vi "Read Status.vi"(8 "error in (no error)":errorcluster, 10 "Source Name (0: Channel 1)":i32(ring) items=["Channel 1", "Channel 2", "Channel 3", "Channel 4", "Common 1", "Common 2", "Differential 1", "Differential 2", "Function 1", "Function 2", "Function 3", "Function 4", "Function 5", "Function 6", "Function 7", "Function 8", "Function 9", "Function 10", "Function 11", "Function 12", "Function 13", "Function 14", "Function 15", "Function 16", "Histogram", "Memory 1", "Memory 2", "Memory 3", "Memory 4", "Clock", "MTRend", "MSPecturm", "Equalized", "Bus 1", "Bus 2", "Bus 3", "Bus 4", "Digital 0", "Digital 1", "Digital 2", "Digital 3", "Digital 4", "Digital 5", "Digital 6", "Digital 7", "Digital 8", "Digital 9", "Digital 10", "Digital 11", "Digital 12", "Digital 13", "Digital 14", "Digital 15", "Pod 1", "Pod 2"], 11 "VISA resource name":refnum<visa-resource-name>) -> (0 "error out":errorcluster, 2 "Source Status (T: ON)":bool=TRUE, 3 "VISA resource name out":refnum<visa-resource-name>)   [LabVIEW 2020, in "Agilent 90000 Series.lvlib"]
doc: "Queries whether the specified channel, function, wmemory, histogram, measurement trend, measurement spectrum, or equalized waveform is on or off."
uses:
  Agilent 90000 Series.lvlib
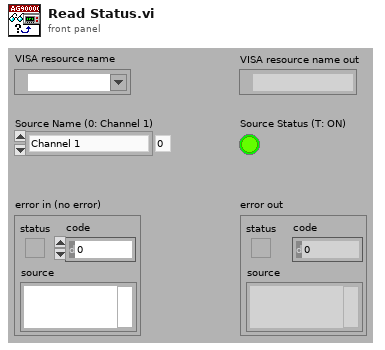
[diagram p1: front panel]
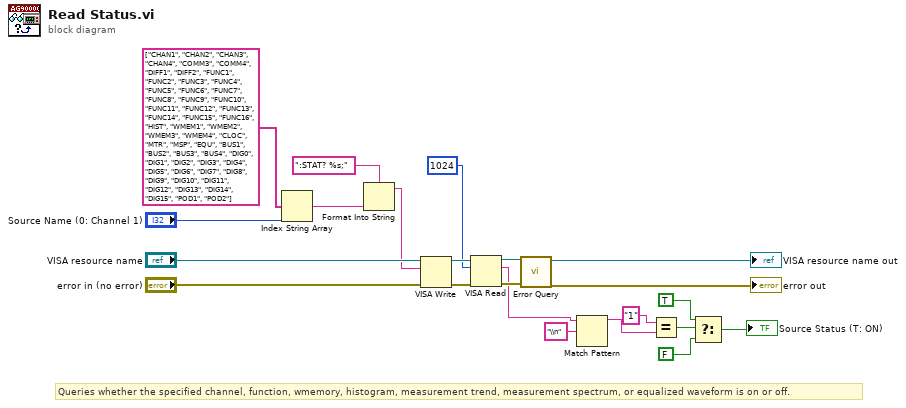
[diagram p0: block diagram]
diagram:
  # "Queries whether the specified channel, function, wmemory, histogram, measurement trend, measurement spectrum, or equalized waveform is on or off."
  n1 = Index String Array(1:"Source Name (0: Channel 1)", 2:string[] ["CHAN1", "CHAN2", "CHAN3", "CHAN4", "COMM3", "COMM4", "DIFF1", "DIFF2", "FUNC1", "FUNC2", "FUNC3", "FUNC4", "FUNC5", "FUNC6", "FUNC7", "FUNC8", "FUNC9", "FUNC10", "FUNC11", "FUNC12", "FUNC13", "FUNC14", "FUNC15", "FUNC16", "HIST", "WMEM1", "WMEM2", "WMEM3", "WMEM4", "CLOC", "MTR", "MSP", "EQU", "BUS1", "BUS2", "BUS3", "BUS4", "DIG0", "DIG1", "DIG2", "DIG3", "DIG4", "DIG5", "DIG6", "DIG7", "DIG8", "DIG9", "DIG10", "DIG11", "DIG12", "DIG13", "DIG14", "DIG15", "POD1", "POD2"] ("string array")) -> (0:w15:string)  [unwired: 1 in]
  n2 = Format Into String(format string=":STAT? %s;", w15) -> (resulting string=w14:string)  [unwired: 2 in, 1 out]
  n3 = VISA Write(VISA resource name="VISA resource name", write buffer=w14, error in (no error)="error in (no error)") -> (VISA resource name out=w13:refnum<visa-resource-name>, error out=w12:errorcluster)  [unwired: 1 out]
  n4 = VISA Read(VISA resource name=w13, byte count=u32 1024, error in (no error)=w12) -> (VISA resource name out=w11:refnum<visa-resource-name>, read buffer=w3:string, error out=w10:errorcluster)  [unwired: 1 out]
  n5 = call "Error Query.vi"("error in (no error)"=w10, "VISA resource name"=w11) -> ("error out"=→"error out":errorcluster, "VISA resource name out"=→"VISA resource name out":refnum<visa-resource-name>)  [unwired: 6 in, 2 out]
  n6 = Match Pattern(string=w3, regular expression="\\n") -> (before substring=w1:string)  [unwired: 1 in, 3 out]
  n7 = Equal?(x="1", y=w1) -> (x = y?=w7:bool)
  n8 = Select(t=TRUE, s=w7, f=FALSE) -> (s? t:f=→"Source Status (T: ON)":bool)
